vi "Build Frame.vi"(7 "measurement configuration":T4 {"FD Baudrate CAN" format="%x"; "Baudrate CAN" format="%x"}, 11 "OOB to Logic Data in":T3 {"Payload LIN" format="%x"; "ID LIN" format="%x"; "Payload CAN" format="%x"; "Type CAN" items=["CAN Data"=0, "CAN Remote"=1, "CAN Bus Error"=2, "CAN 2.0 Data"=8, "CAN FD Data"=16, "CAN FD+BRS Data"=24, "J1939 Data"=192, "Delay"=224, "Log Trigger"=225, "Start Trigger"=226]; "ID CAN" format="%x"}) -> (2 "DLC out":u32, 3 "output cluster":T1 {"payload" format="%x"; "timestamp" format="%<%.7X\n%x>T"; "type" items=["CAN Data"=0, "CAN Remote"=1, "CAN Bus Error"=2, "CAN 2.0 Data"=8, "CAN FD Data"=16, "CAN FD+BRS Data"=24, "J1939 Data"=192, "Delay"=224, "Log Trigger"=225, "Start Trigger"=226]; "identifier" format="%x"})   [LabVIEW 2025, in "CAN-LIN Frame Generator.lvclass"]
uses:
  CAN-LIN Frame Generator.lvclass
  Measurement Configuration.ctl
  CAN-LIN Frame Generator UI/Toggle.ctl
  OOB Data Transfer/Typdefs/OOB to Logic Data.ctl
  <vilib>/xnet/xnet.llb/XNET Frame Type CAN.ctl
  <vilib>/xnet/xnet.llb/XNET Frame CAN.ctl
  CAN-LIN Frame Generator.lvclass/CAN-LIN Frame Generator.ctl
  OOB Data Transfer/OOB Data Transfer.lvlib
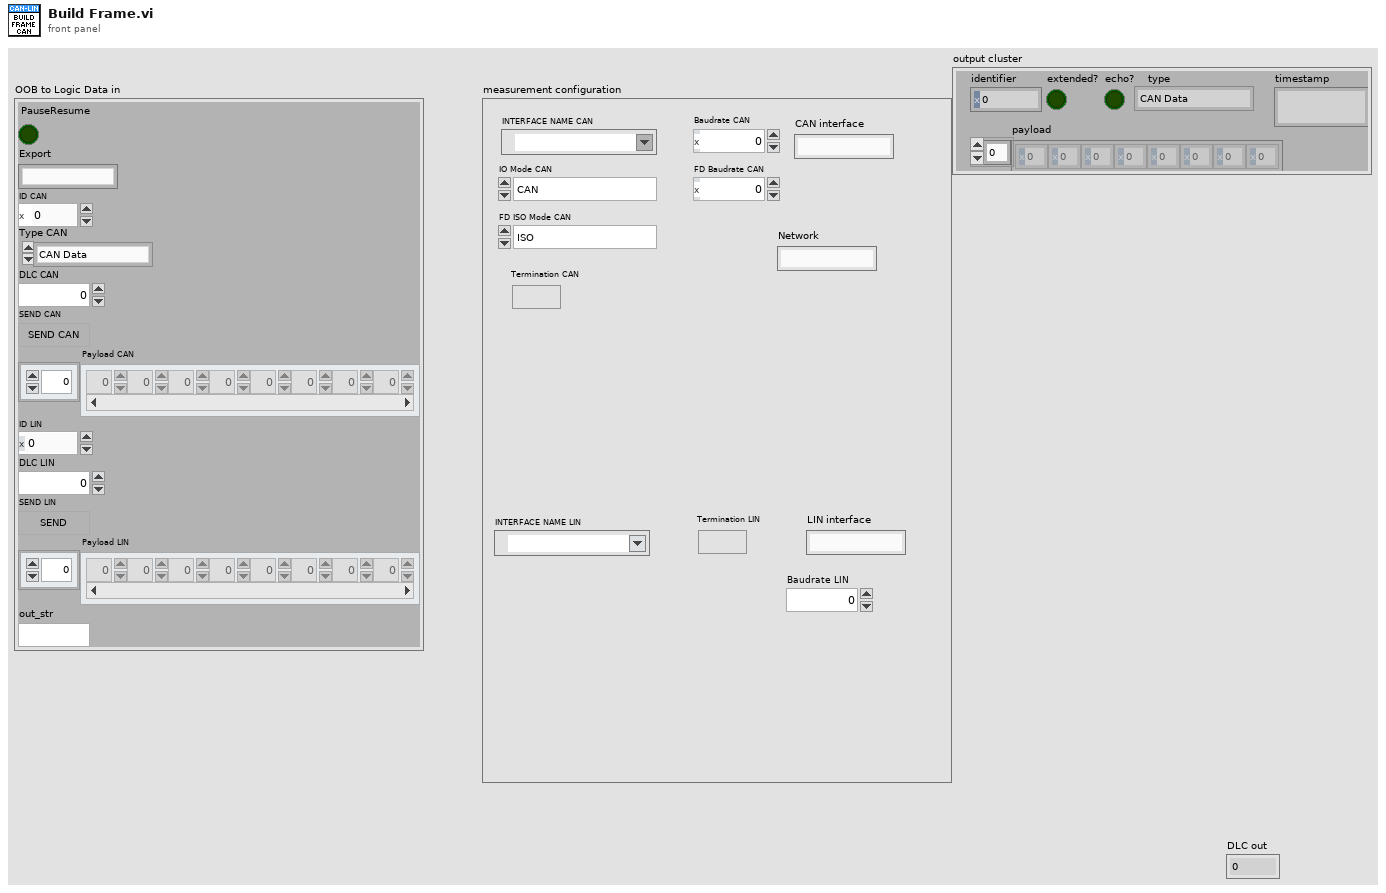
[diagram p1: front panel]
types:
  T1 = typedef "XNET Frame CAN.ctl" = cluster{"timestamp":timestamp, "payload":u8[], "identifier":u32, "type":T2, "extended?":bool, "echo?":bool}
  T2 = typedef "XNET Frame Type CAN.ctl" = u8
  T3 = typedef "OOB Data Transfer.lvlib/OOB to Logic Data.ctl" = cluster{"PauseResume":bool, "Export":string, "ID CAN":u32, "Type CAN":T2, "DLC CAN":u32, "SEND CAN":bool, "Payload CAN":u32[], "ID LIN":u32, "DLC LIN":u32, "SEND LIN":bool, "Payload LIN":u32[], "out_str":string}
  T4 = typedef "CAN-LIN Frame Generator.lvclass/Measurement Configuration.ctl" = cluster{"INTERFACE NAME CAN":refnum<k21>, "IO Mode CAN":enum32{"CAN", "CAN FD", "CAN FD + BRS"}, "FD ISO Mode CAN":enum32{"ISO", "Legacy ISO", "Non-ISO"}, "Termination CAN":T5, "Baudrate CAN":u32, "FD Baudrate CAN":u32, "INTERFACE NAME LIN":refnum<k21>, "Termination LIN":T5, "CAN interface":string, "LIN interface":string, "Network":string, "Baudrate LIN":u32}
  T5 = typedef "Toggle.ctl" = bool
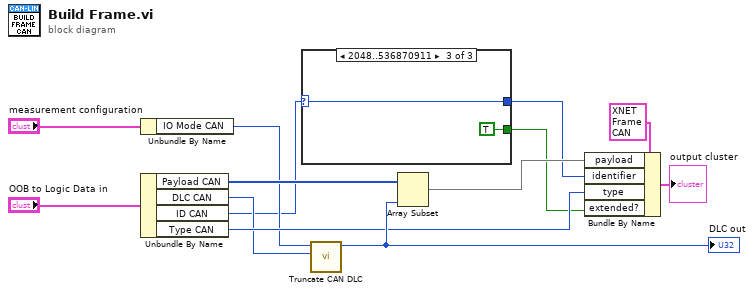
[diagram p0: block diagram]
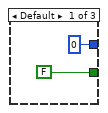
[diagram p2: hidden frame]
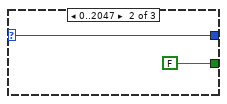
[diagram p3: hidden frame]
diagram:
  n1 = Unbundle By Name("measurement configuration") -> ("IO Mode CAN"=w6:enum32{"CAN", "CAN FD", "CAN FD + BRS"})
  n2 = Unbundle By Name("OOB to Logic Data in") -> ("Payload CAN"=w8:u32[], "DLC CAN"=w5:u32, "ID CAN"=w4:u32, "Type CAN"=w7:T2)
  n3 = case shown="2048..536870911" w4 {
    selector: w4 -> [_ w17 w19]
    tunnel: [u32 0 ("ID CAN") w17 w19] -> w3
    tunnel: [FALSE FALSE TRUE] -> w1
    frame Default {
    }
    frame 0..2047 {
    }
    frame 2048..536870911 {
    }
  }
  n4 = call "Truncate CAN DLC.vi"("DLC in"=w5, "IO Mode"=w6) -> ("DLC out"=w10:u32)  [unwired: 9 in]
  "DLC out" <- w10
  n5 = Array Subset(array=w8, length=w10) -> (w9:u32[])  [unwired: 1 in]
  n6 = Bundle By Name(cluster=T1 {"timestamp"=timestamp(0 s since 1904-01-01), "payload"=[], "identifier"=123, "type"=0, "extended?"=TRUE, "echo?"=FALSE} ("CAN frame"), "payload"=w9, "identifier"=w3, "type"=w7, "extended?"=w1) -> (→"output cluster":T1)
